vi "AH Bridge Check RTC and Set.vi"(8 "error in (no error)":errorcluster {"code" format="%.0x"}, 11 "VISA resource name":refnum<visa-resource-name>) -> (0 "error out":errorcluster {"code" format="%.0x"}, 1 "Time Not Correct":bool, 2 "Date Not Correct":bool, 3 "dup VISA Session":refnum<visa-resource-name>)   [LabVIEW 2025]
doc: "This VI reads the real time clock (RTC) and sets the clock if it varies from the current date and time\nScott Hannahs <sth@magnet.fsu.edu>\nAuthor: Scott Hannahs <sth@magnet.fsu.edu>\n\nThis software is licensed for use under the “MIT License\"\nCopyright (c) 2025 Scott Hannahs, sth@sth@magnet.sthnet.net\n\nPermission is hereby granted, free of charge, to any person obtaining a copy of this software and associated documentation files (the \"Software\"), to deal in the Software without restriction, including without limitation the rights to use, copy, modify, merge, publish, distribute, sublicense, and/or sell copies of the Software, and to permit persons to whom the Software is furnished to do so, subject to the following conditions: The above copyright notice and this permission notice shall be included in all copies or substantial portions of the Software.\n\nTHE SOFTWARE IS PROVIDED \"AS IS\", WITHOUT WARRANTY OF ANY KIND, EXPRESS OR IMPLIED, INCLUDING BUT NOT LIMITED TO THE WARRANTIES OF MERCHANTABILITY, FITNESS FOR A PARTICULAR PURPOSE AND NONINFRINGEMENT. IN NO EVENT SHALL THE AUTHORS OR COPYRIGHT HOLDERS BE LIABLE FOR ANY CLAIM, DAMAGES OR OTHER LIABILITY, WHETHER IN AN ACTION OF CONTRACT, TORT OR OTHERWISE, ARISING FROM, OUT OF OR IN CONNECTION WITH THE SOFTWARE OR THE USE OR OTHER DEALINGS IN THE SOFTWARE."
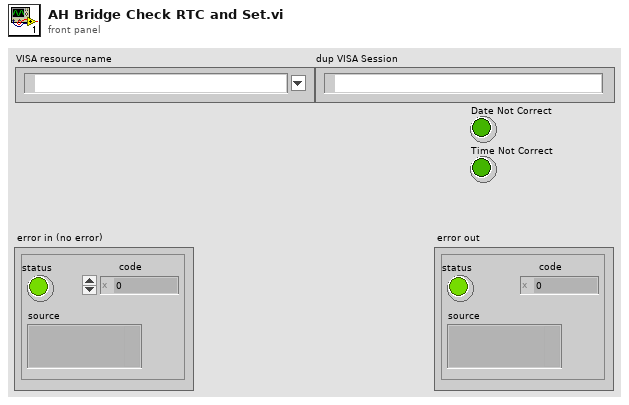
[diagram p1: front panel]
types:
  T1 = typedef "LVDateTimeRec.ctl" = cluster{"fractional second":dbl, "second":i32, "minute":i32, "hour":i32, "day of month":i32, "month":i32, "year":i32, "day of week":i32, "day of year":i32, "DST":i32}
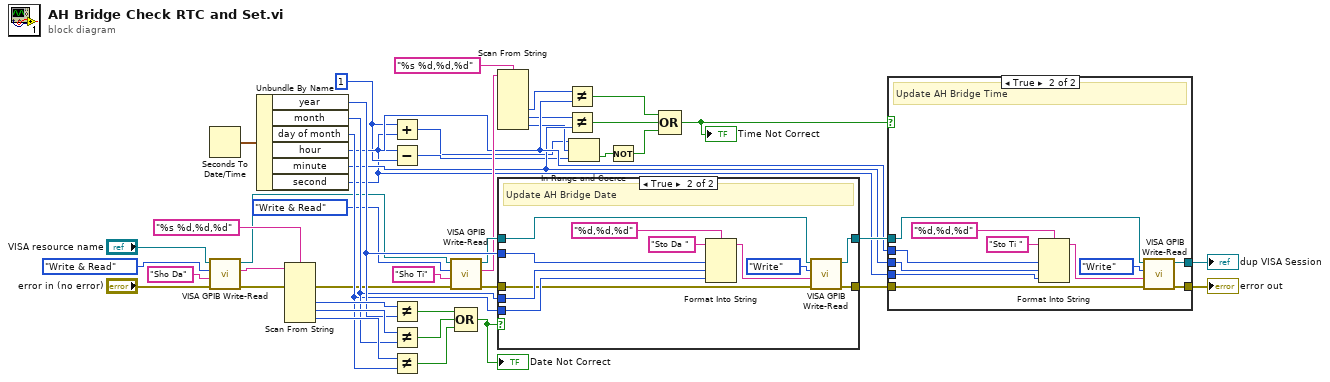
[diagram p0: block diagram]
diagram:
  w5 = 1 ("x")
  n1 = Seconds To Date/Time() -> (date time rec=w37:T1)  [unwired: 2 in]
  n2 = call "VISA GPIB Write-Read.vi"("error in (no error)"="error in (no error)", "Command"="Sho Da", "Action"=enum16{"Write", "Read", "Write & Read"}."Write & Read", "VISA resource name"="VISA resource name") -> ("error out"=w39:errorcluster, "String Returned"=w42:string, "dup VISA Session"=w24:refnum<visa-resource-name>)  [unwired: 4 in, 1 out]
  n3 = Unbundle By Name(w37) -> ("year"=w29:i32, "month"=w28:i32, "day of month"=w27:i32, "hour"=w10:i32, "minute"=w7:i32, "second"=w4:i32)
  n4 = Scan From String(format string="%s %d,%d,%d", input string=w42, error in=w39) -> (error out=w16:errorcluster, output 2=w31:i32, output 3=w32:i32, output 4=w33:i32)  [unwired: 6 in, 2 out]
  n5 = Add(x=w5, y=w4) -> (x+y=w2:i32)
  n6 = Subtract(x=w4, y=w5) -> (x-y=w3:i32)
  n7 = Not Equal?(x=w31, y=w29) -> (x != y?=w36:bool)
  n8 = Not Equal?(x=w32, y=w28) -> (x != y?=w35:bool)
  n9 = Not Equal?(x=w33, y=w27) -> (x != y?=w34:bool)
  n10 = call "VISA GPIB Write-Read.vi"("error in (no error)"=w16, "Command"="Sho Ti", "Action"=enum16{"Write", "Read", "Write & Read"}."Write & Read", "VISA resource name"=w24) -> ("error out"=w15:errorcluster, "String Returned"=w18:string, "dup VISA Session"=w23:refnum<visa-resource-name>)  [unwired: 4 in, 1 out]
  n11 = Compound Arithmetic op=OR(w36, w35, w34) -> (w30:bool)
  "Date Not Correct" <- w30
  n12 = Scan From String(format string="%s %d,%d,%d", input string=w18) -> (output 2=w17:i32, output 3=w9:i32, output 4=w6:i32)  [unwired: 7 in, 3 out]
  n13 = case shown="True" w30 {
    tunnel: w29 -> [_ w55]
    tunnel: w28 -> [_ w54]
    tunnel: w27 -> [_ w53]
    tunnel: w23 -> [w46 w52]
    tunnel: [w46 w51] -> w12
    tunnel: w15 -> [w45 w49]
    tunnel: [w45 w50] -> w14
    frame False {
      # "AH Bridge Date is Correct"
    }
    frame True {
      # "Update AH Bridge Date"
      n14 = Format Into String(format string="%d,%d,%d", initial string="Sto Da ", w55, w54, w53) -> (resulting string=w47:string)  [unwired: 1 in, 1 out]
      n15 = call "VISA GPIB Write-Read.vi"("error in (no error)"=w49, "Command"=w47, "Action"=enum16{"Write", "Read", "Write & Read"}."Write", "VISA resource name"=w52) -> ("error out"=w50:errorcluster, "dup VISA Session"=w51:refnum<visa-resource-name>)  [unwired: 4 in, 2 out]
    }
  }
  n16 = Not Equal?(x=w17, y=w10) -> (x != y?=w20:bool)
  n17 = Not Equal?(x=w9, y=w7) -> (x != y?=w21:bool)
  n18 = In Range and Coerce(upper limit=w2, x=w6, lower limit=w3) -> (In Range?=w22:bool)  [unwired: 1 out]
  n19 = Not(x=w22) -> (.not. x?=w1:bool)
  n20 = Compound Arithmetic op=OR(w20, w21, w1) -> (w8:bool)
  "Time Not Correct" <- w8
  n21 = case shown="True" w8 {
    tunnel: w14 -> [w59 w63]
    tunnel: [w59 w65] -> w13
    tunnel: w12 -> [w58 w64]
    tunnel: [w58 w66] -> w11
    tunnel: w10 -> [_ w62]
    tunnel: w7 -> [_ w61]
    tunnel: w4 -> [_ w60]
    frame False {
      # "AH Bridge Time is Correct"
    }
    frame True {
      # "Update AH Bridge Time"
      n22 = Format Into String(format string="%d,%d,%d", initial string="Sto Ti ", w62, w61, w60) -> (resulting string=w70:string)  [unwired: 1 in, 1 out]
      n23 = call "VISA GPIB Write-Read.vi"("error in (no error)"=w63, "Command"=w70, "Action"=enum16{"Write", "Read", "Write & Read"}."Write", "VISA resource name"=w64) -> ("error out"=w65:errorcluster, "dup VISA Session"=w66:refnum<visa-resource-name>)  [unwired: 4 in, 2 out]
    }
  }
  "dup VISA Session" <- w11
  "error out" <- w13
